vi "HFRR ADV v04 new software.vi"() -> ()   [LabVIEW 2025] (continued)
                  n3123 = local write "S 98"(w4157) -> ()
                }
                frame 97 {
                  n3124 = local write "S 99"(w4158) -> ()
                }
                frame 98 {
                  n3125 = local write "S 100"(w4159) -> ()
                }
                frame 99 {
                  n3126 = local write "S 101"(w4160) -> ()
                }
                frame 100 {
                  n3127 = local write "S 102"(w4161) -> ()
                }
                frame 101 {
                  n3128 = local write "S 103"(w4162) -> ()
                }
                frame 102 {
                  n3129 = local write "S 104"(w4163) -> ()
                }
                frame 103 {
                  n3130 = local write "S 105"(w4164) -> ()
                }
                frame 104 {
                  n3131 = local write "S 106"(w4165) -> ()
                }
                frame 105 {
                }
                frame 106 {
                  n3132 = property on="OK Button 17" class="Bool (strict)"("Boolean Text.Text"=w4166) -> ()  [unwired: 2 in, 2 out]
                }
                frame 107 {
                  n3133 = property on="OK Button 16" class="Bool (strict)"("Boolean Text.Text"=w4167) -> ()  [unwired: 2 in, 2 out]
                }
                frame 108 {
                  n3134 = property on="TITTLE" class="Str"("Caption.Text"=w4168) -> ()  [unwired: 2 in, 2 out]
                }
                frame 109 {
                  "String 30" <- w4169
                }
                frame 110 {
                  n3135 = property on="Test Date" class="Str"("Caption.Text"=w4170) -> ()  [unwired: 2 in, 2 out]
                  "String 31" <- w4170
                }
                frame 111 {
                  n3136 = property on="Sample ID" class="Str"("Caption.Text"=w4171) -> ()  [unwired: 2 in, 2 out]
                  "String 32" <- w4171
                }
                frame 112 {
                  n3137 = property on="Tested by" class="Str"("Caption.Text"=w4172) -> ()  [unwired: 2 in, 2 out]
                  "String 33" <- w4172
                }
                frame 113 {
                  n3138 = property on="System Configured Printers 2" class="Arr (strict)"("Caption.Text"=w4173) -> ()  [unwired: 2 in, 2 out]
                }
                frame 114 {
                  n3139 = property on="Selected Printer" class="Str"("Caption.Text"=w4174) -> ()  [unwired: 2 in, 2 out]
                }
                frame 115 {
                  n3140 = property on="Select Printer 3" class="DigNum (strict)"("Caption.Text"=w4175) -> ()  [unwired: 2 in, 2 out]
                }
                frame 116 {
                  n3141 = property on="Print" class="Bool (strict)"("Boolean Text.Text"=w4176) -> ()  [unwired: 2 in, 2 out]
                }
                frame 117 {
                  "String 41" <- w4177
                }
                frame 118 {
                  n3142 = property on="tested by" class="Str"("Caption.Text"=w4178) -> ()  [unwired: 2 in, 2 out]
                }
                frame 119 {
                }
                frame 120 {
                  n3143 = property on="Export" class="Bool (strict)"("Boolean Text.Text"=w4179) -> ()  [unwired: 2 in, 2 out]
                }
                frame 121 {
                  n3144 = property on="TEMP INTERCEPT:" class="DigNum (strict)"("Caption.Text"=w4180) -> ()  [unwired: 2 in, 2 out]
                }
                frame 122 {
                  n3145 = property on="AIR TEMP INTERCEPT:" class="DigNum (strict)"("Caption.Text"=w4181) -> ()  [unwired: 2 in, 2 out]
                }
                frame 123 {
                  n3146 = property on="Select File Type" class="Enum (strict)"("Caption.Text"=w4182) -> ()  [unwired: 2 in, 2 out]
                }
                frame 124 {
                  n3147 = property on="s.NO" class="Str"("Caption.Text"=w4183) -> ()  [unwired: 2 in, 2 out]
                  "String 45" <- w4183
                }
                frame 125 {
                  n3148 = property on="trip1 8" class="Bool (strict)"("Boolean Text.Text"=w4184) -> ()  [unwired: 2 in, 2 out]
                }
                frame 126, Default {
                }
              }
            }
          }
          frame #1 {
            w4192 = TRUE ("Visible")
            n3149 = local read "S 91"() -> (w4209:string)
            n3150 = local read "S 90"() -> (w4208:string)
            n3151 = local read "S 88"() -> (w4207:string)
            n3152 = property on="File Path" class="Path"("Caption.Text"=w4208) -> ()  [unwired: 2 in, 2 out]
            n3153 = property on="SrvM CP" class="Bool (strict)"("Boolean Text.Text"=w4207) -> ()  [unwired: 2 in, 2 out]
            n3154 = local read "S 71"() -> (w4202:string)
            n3155 = local read "S 86"() -> (w4204:string)
            n3156 = local read "S 85"() -> (w4205:string)
            n3157 = local read "S 87"() -> (w4203:string)
            n3158 = local read "S 84"() -> (w4206:string)
            n3159 = local read "S 103"() -> (w4191:string)
            n3160 = local read "S 104"() -> (w4190:string)
            n3161 = property on="ENTER THE NEW PASSWORD" class="Str"("Caption.Text"=w4203) -> ()  [unwired: 2 in, 2 out]
            n3162 = property on="Password" class="Str"("Caption.Text"=w4205) -> ()  [unwired: 2 in, 2 out]
            n3163 = property on="ENTER CURRENT PASSWORD" class="Str"("Caption.Text"=w4204) -> ()  [unwired: 2 in, 2 out]
            n3164 = property on="EDIT" class="Bool (strict)"("Boolean Text.Text"=w4202) -> ()  [unwired: 2 in, 2 out]
            n3165 = property on="SAVE" class="Bool (strict)"("Boolean Text.Text"=w4206) -> ()  [unwired: 2 in, 2 out]
            n3166 = Build Array(w4191, w4190) -> (w4189:string[])
            n3167 = property on="Heater Button" class="Bool (strict)"("Strings [4]"=w4189) -> ()  [unwired: 2 in, 2 out]
            n3168 = property on="CH-HUMIDITY WET" class="DigNum (strict)"("Caption.Size to Text?"=w4192) -> ()  [unwired: 2 in, 2 out]
            n3169 = property on="CH-HUMIDITY DRY" class="DigNum (strict)"("Caption.Size to Text?"=w4192) -> ()  [unwired: 2 in, 2 out]
            n3170 = property on="CH-POWER -" class="DigNum (strict)"("Caption.Size to Text?"=w4192) -> ()  [unwired: 2 in, 2 out]
            n3171 = property on="CH-HEATER" class="DigNum (strict)"("Caption.Size to Text?"=w4192) -> ()  [unwired: 2 in, 2 out]
            n3172 = property on="CH-POWER +" class="DigNum (strict)"("Caption.Size to Text?"=w4192) -> ()  [unwired: 2 in, 2 out]
            n3173 = local read "S 92"() -> (w4201:string)
            n3174 = local read "S 93"() -> (w4200:string)
            n3175 = local read "S 105"() -> (w4187:string)
            n3176 = local read "S 106"() -> (w4186:string)
            n3177 = Build Array(w4201, w4200) -> ()  [unwired: 1 out]
            n3178 = Build Array(w4187, w4186) -> (w4188:string[])
            n3179 = local read "S 95"() -> (w4198:string)
            n3180 = local read "S 94"() -> (w4199:string)
            n3181 = local read "bs"() -> (w4214:string)
            n3182 = local read "as"() -> (w4215:string)
            n3183 = property on="Humidity" class="Bool (strict)"("Strings [4]"=w4188) -> ()  [unwired: 2 in, 2 out]
            n3184 = Concatenate Strings(w4214, "\r", w4215) -> ()  [unwired: 1 out]
            n3185 = property on="STROKE GAIN :" class="DigNum (strict)"("Caption.Text"=w4198) -> ()  [unwired: 2 in, 2 out]
            n3186 = property on="DISPLACEMENT :" class="DigNum (strict)"("Caption.Text"=w4199) -> ()  [unwired: 2 in, 2 out]
            n3187 = property on="Rh After" class="DigNum (strict)"("Caption.Size to Text?"=TRUE ("Caption.Size to Text")) -> ()  [unwired: 2 in, 2 out]
            n3188 = local read "S 48"() -> (w4238:string)
            n3189 = local read "S 50"() -> (w4236:string)
            n3190 = local read "S 51"() -> (w4235:string)
            n3191 = local read "S 49"() -> (w4237:string)
            n3192 = local read "S 52"() -> (w4234:string)
            n3193 = local read "as"() -> (w4219:string)
            n3194 = local read "bs"() -> (w4220:string)
            n3195 = local read "S 56"() -> (w4233:string)
            n3196 = local read "S 57"() -> (w4232:string)
            n3197 = local read "S 58"() -> (w4231:string)
            n3198 = local read "S 59"() -> (w4230:string)
            n3199 = property on="OPEN" class="Bool (strict)"("Boolean Text.Text"=w4234) -> ()  [unwired: 2 in, 2 out]
            n3200 = property on="OPEN 1" class="Bool (strict)"("Boolean Text.Text"=w4238) -> ()  [unwired: 2 in, 2 out]
            n3201 = property on="OPEN 2" class="Bool (strict)"("Boolean Text.Text"=w4237) -> ()  [unwired: 2 in, 2 out]
            n3202 = property on="OPEN 3" class="Bool (strict)"("Boolean Text.Text"=w4236) -> ()  [unwired: 2 in, 2 out]
            n3203 = property on="OPEN 4" class="Bool (strict)"("Boolean Text.Text"=w4235) -> ()  [unwired: 2 in, 2 out]
            n3204 = Concatenate Strings(w4220, "\r", w4219) -> ()  [unwired: 1 out]
            n3205 = local read "S 102"() -> (w4193:string)
            n3206 = property on="КОФ1" class="DigNum (strict)"("Caption.Text"=w4233) -> ()  [unwired: 2 in, 2 out]
            n3207 = local read "S 98"() -> (w4197:string)
            n3208 = local read "S 99"() -> (w4196:string)
            n3209 = local read "S 100"() -> (w4195:string)
            n3210 = local read "S 101"() -> (w4194:string)
            n3211 = property on="КОФ2" class="DigNum (strict)"("Caption.Text"=w4232) -> ()  [unwired: 2 in, 2 out]
            n3212 = property on="КОФ3" class="DigNum (strict)"("Caption.Text"=w4231) -> ()  [unwired: 2 in, 2 out]
            n3213 = property on="КОФ4" class="DigNum (strict)"("Caption.Text"=w4230) -> ()  [unwired: 2 in, 2 out]
            n3214 = local read "bs"() -> (w4218:string)
            n3215 = local read "as"() -> (w4217:string)
            n3216 = property on="CH-POWER +" class="DigNum (strict)"("Caption.Text"=w4197) -> ()  [unwired: 2 in, 2 out]
            n3217 = property on="CH-POWER -" class="DigNum (strict)"("Caption.Text"=w4196) -> ()  [unwired: 2 in, 2 out]
            n3218 = property on="CH-HEATER" class="DigNum (strict)"("Caption.Text"=w4195) -> ()  [unwired: 2 in, 2 out]
            n3219 = property on="CH-HUMIDITY DRY" class="DigNum (strict)"("Caption.Text"=w4194) -> ()  [unwired: 2 in, 2 out]
            n3220 = property on="CH-HUMIDITY WET" class="DigNum (strict)"("Caption.Text"=w4193) -> ()  [unwired: 2 in, 2 out]
            n3221 = local read "S 60"() -> (w4229:string)
            n3222 = local read "S 54"() -> (w4239:string)
            n3223 = Concatenate Strings(w4218, "\r", w4217) -> ()  [unwired: 1 out]
            n3224 = Concatenate Strings(w4239, w4229) -> ()  [unwired: 1 out]
            n3225 = local read "S 77"() -> (→"String 43":string)
            n3226 = local read "S 76"() -> (w4212:string)
            n3227 = local read "S 78"() -> (w4211:string)
            n3228 = local read "S 71"() -> (w4223:string)
            n3229 = local read "S 66"() -> (w4228:string)
            n3230 = local read "S 67"() -> (w4227:string)
            n3231 = local read "S 68"() -> (w4226:string)
            n3232 = local read "S 69"() -> (w4225:string)
            n3233 = local read "S 70"() -> (w4224:string)
            n3234 = property on="AIR TEMP" class="DigNum (strict)"("Caption.Text"=w4211) -> ()  [unwired: 2 in, 2 out]
            n3235 = property on="Set Strk" class="DigNum (strict)"("Caption.Text"=w4212) -> ()  [unwired: 2 in, 2 out]
            n3236 = property on="FRIC. FORCE :" class="DigNum (strict)"("Caption.Text"=w4228) -> ()  [unwired: 2 in, 2 out]
            n3237 = property on="TEMPERATURE :" class="DigNum (strict)"("Caption.Text"=w4227) -> ()  [unwired: 2 in, 2 out]
            n3238 = property on="SPEED OUT:" class="DigNum (strict)"("Caption.Text"=w4226) -> ()  [unwired: 2 in, 2 out]
            n3239 = property on="AIR TEMPERATURE :" class="DigNum (strict)"("Caption.Text"=w4225) -> ()  [unwired: 2 in, 2 out]
            n3240 = property on="HUMIDITY:" class="DigNum (strict)"("Caption.Text"=w4224) -> ()  [unwired: 2 in, 2 out]
            n3241 = property on="EDIT" class="Bool (strict)"("Boolean Text.Text"=w4223) -> ()  [unwired: 2 in, 2 out]
            n3242 = local read "S 79"() -> (w4210:string)
          }
          frame #2 {
          }
        }
        n3243 = local write "Lan flag"(10.0 ("Lan flag")) -> ()
      }
      frame Enabled {
      }
    }
    n3244 = Wait (ms)(milliseconds to wait=u32 2000) -> ()  [unwired: 1 out]
    n3245 = local read "Quit"() -> (w4013:bool)
  }
  n3246 = disable-structure shown="Disabled" {
    frame Disabled {
      n3247 = while {
        tunnel: [w4241] -> _
        i -> [w4241]
        stop <- w4240 continue-if-true
        n3248 = Wait (ms)(milliseconds to wait=u32 50) -> ()  [unwired: 1 out]
        n3249 = stacked-sequence {
          frame #0 {
            # "Controls Text color"
            # "Controls BG color"
            n3250 = property on="FILE" class="Str"("Text.Text Colors:Text Color"="SC  Text") -> ()  [unwired: 2 in, 2 out]
            n3251 = property on="Fuel Discription :" class="Str"("Text.Text Colors:Text Color"="SC  Text") -> ()  [unwired: 2 in, 2 out]
            n3252 = property on="tested by" class="Str"("Text.Text Colors:Text Color"="SC  Text") -> ()  [unwired: 2 in, 2 out]
            n3253 = property on="Remarks :" class="Str"("Text.Text Colors:Text Color"="SC  Text") -> ()  [unwired: 2 in, 2 out]
            n3254 = property class="DigNum (strict)"("Numeric Text.Text Colors:BG Color"="NC BG") -> ()  [unwired: 2 in, 2 out]
            n3255 = property class="DigNum (strict)"("Numeric Text.Text Colors:BG Color"="NC BG") -> ()  [unwired: 2 in, 2 out]
            n3256 = property class="DigNum (strict)"("Numeric Text.Text Colors:BG Color"="NC BG") -> ()  [unwired: 2 in, 2 out]
            n3257 = property class="DigNum (strict)"("Numeric Text.Text Colors:BG Color"="NC BG") -> ()  [unwired: 2 in, 2 out]
            n3258 = property class="DigNum (strict)"("Numeric Text.Text Colors:BG Color"="NC BG") -> ()  [unwired: 2 in, 2 out]
            n3259 = property class="DigNum (strict)"("Numeric Text.Text Colors:BG Color"="NC BG") -> ()  [unwired: 2 in, 2 out]
            n3260 = property class="DigNum (strict)"("Numeric Text.Text Colors:BG Color"="NC BG") -> ()  [unwired: 2 in, 2 out]
            n3261 = property class="DigNum (strict)"("Numeric Text.Text Colors:BG Color"="NC BG") -> ()  [unwired: 2 in, 2 out]
            n3262 = property class="DigNum (strict)"("Numeric Text.Text Colors:BG Color"="NC BG") -> ()  [unwired: 2 in, 2 out]
            n3263 = property class="DigNum (strict)"("Numeric Text.Text Colors:BG Color"="NC BG") -> ()  [unwired: 2 in, 2 out]
            n3264 = property class="DigNum (strict)"("Numeric Text.Text Colors:BG Color"="NC BG") -> ()  [unwired: 2 in, 2 out]
            n3265 = property class="DigNum (strict)"("Numeric Text.Text Colors:BG Color"="NC BG") -> ()  [unwired: 2 in, 2 out]
            n3266 = property on="FILE" class="Str"("Text.Text Colors:BG Color"="SC BG 3") -> ()  [unwired: 2 in, 2 out]
            n3267 = property on="Fuel Discription :" class="Str"("Text.Text Colors:BG Color"="SC BG 3") -> ()  [unwired: 2 in, 2 out]
            n3268 = property on="tested by" class="Str"("Text.Text Colors:BG Color"="SC BG 3") -> ()  [unwired: 2 in, 2 out]
            n3269 = property on="Remarks :" class="Str"("Text.Text Colors:BG Color"="SC BG 3") -> ()  [unwired: 2 in, 2 out]
            n3270 = property class="DigNum (strict)"("Numeric Text.Text Colors:Text Color"="NC Text") -> ()  [unwired: 2 in, 2 out]
            n3271 = property class="DigNum (strict)"("Numeric Text.Text Colors:Text Color"="NC Text") -> ()  [unwired: 2 in, 2 out]
            n3272 = property class="DigNum (strict)"("Numeric Text.Text Colors:Text Color"="NC Text") -> ()  [unwired: 2 in, 2 out]
            n3273 = property class="DigNum (strict)"("Numeric Text.Text Colors:Text Color"="NC Text") -> ()  [unwired: 2 in, 2 out]
            n3274 = property class="DigNum (strict)"("Numeric Text.Text Colors:Text Color"="NC Text") -> ()  [unwired: 2 in, 2 out]
            n3275 = property class="DigNum (strict)"("Numeric Text.Text Colors:Text Color"="NC Text") -> ()  [unwired: 2 in, 2 out]
            n3276 = property class="DigNum (strict)"("Numeric Text.Text Colors:Text Color"="NC Text") -> ()  [unwired: 2 in, 2 out]
            n3277 = property class="DigNum (strict)"("Numeric Text.Text Colors:Text Color"="NC Text") -> ()  [unwired: 2 in, 2 out]
            n3278 = property class="DigNum (strict)"("Numeric Text.Text Colors:Text Color"="NC Text") -> ()  [unwired: 2 in, 2 out]
            n3279 = property class="DigNum (strict)"("Numeric Text.Text Colors:Text Color"="NC Text") -> ()  [unwired: 2 in, 2 out]
            n3280 = property class="DigNum (strict)"("Numeric Text.Text Colors:Text Color"="NC Text") -> ()  [unwired: 2 in, 2 out]
            n3281 = property class="DigNum (strict)"("Numeric Text.Text Colors:Text Color"="NC Text") -> ()  [unwired: 2 in, 2 out]
            n3282 = property class="DigNum (strict)"("Numeric Text.Text Colors:Text Color"="NI Text  2") -> ()  [unwired: 2 in, 2 out]
            n3283 = property class="DigNum (strict)"("Numeric Text.Text Colors:Text Color"="NI Text  2") -> ()  [unwired: 2 in, 2 out]
            n3284 = property class="DigNum (strict)"("Numeric Text.Text Colors:Text Color"="NI Text  2") -> ()  [unwired: 2 in, 2 out]
            n3285 = property class="DigNum (strict)"("Numeric Text.Text Colors:Text Color"="NI Text  2") -> ()  [unwired: 2 in, 2 out]
            n3286 = property class="DigNum (strict)"("Numeric Text.Text Colors:Text Color"="NI Text  2") -> ()  [unwired: 2 in, 2 out]
            n3287 = property class="DigNum (strict)"("Numeric Text.Text Colors:Text Color"="NI Text  2") -> ()  [unwired: 2 in, 2 out]
            n3288 = property class="DigNum (strict)"("Numeric Text.Text Colors:Text Color"="NI Text  2") -> ()  [unwired: 2 in, 2 out]
            n3289 = property class="DigNum (strict)"("Numeric Text.Text Colors:Text Color"="NI Text  2") -> ()  [unwired: 2 in, 2 out]
            n3290 = property class="DigNum (strict)"("Numeric Text.Text Colors:Text Color"="NI Text  2") -> ()  [unwired: 2 in, 2 out]
            n3291 = property class="DigNum (strict)"("Numeric Text.Text Colors:Text Color"="NI Text  2") -> ()  [unwired: 2 in, 2 out]
            n3292 = property class="DigNum (strict)"("Numeric Text.Text Colors:Text Color"="NI Text  2") -> ()  [unwired: 2 in, 2 out]
            n3293 = property class="DigNum (strict)"("Numeric Text.Text Colors:Text Color"="NI Text  2") -> ()  [unwired: 2 in, 2 out]
            n3294 = property class="DigNum (strict)"("Numeric Text.Text Colors:Text Color"="NI Text  2") -> ()  [unwired: 2 in, 2 out]
            n3295 = property class="DigNum (strict)"("Numeric Text.Text Colors:Text Color"="NI Text  2") -> ()  [unwired: 2 in, 2 out]
            n3296 = property class="DigNum (strict)"("Numeric Text.Text Colors:Text Color"="NI Text  2") -> ()  [unwired: 2 in, 2 out]
            n3297 = property on="Coefficient Of Friction" class="XYGraph (strict)"("Plot Area:Colors:FG Color"="GFG  2", "Plot Area:Colors:BG Color"="GBG   2") -> ()  [unwired: 2 in, 2 out]
            n3298 = property on="Humidity ( %RH )" class="XYGraph (strict)"("Plot Area:Colors:FG Color"="GFG  2", "Plot Area:Colors:BG Color"="GBG   2") -> ()  [unwired: 2 in, 2 out]
            n3299 = property on="Air Temperature  ( °C )" class="XYGraph (strict)"("Plot Area:Colors:FG Color"="GFG  2", "Plot Area:Colors:BG Color"="GBG   2") -> ()  [unwired: 2 in, 2 out]
            n3300 = property on="Sample Temperature ( °C )" class="XYGraph (strict)"("Plot Area:Colors:FG Color"="GFG  2", "Plot Area:Colors:BG Color"="GBG   2") -> ()  [unwired: 2 in, 2 out]
            n3301 = property class="DigNum (strict)"("Numeric Text.Text Colors:BG Color"="NI BG 2") -> ()  [unwired: 2 in, 2 out]
            n3302 = property class="DigNum (strict)"("Numeric Text.Text Colors:BG Color"="NI BG 2") -> ()  [unwired: 2 in, 2 out]
            n3303 = property class="DigNum (strict)"("Numeric Text.Text Colors:BG Color"="NI BG 2") -> ()  [unwired: 2 in, 2 out]
            n3304 = property class="DigNum (strict)"("Numeric Text.Text Colors:BG Color"="NI BG 2") -> ()  [unwired: 2 in, 2 out]
            n3305 = property class="DigNum (strict)"("Numeric Text.Text Colors:BG Color"="NI BG 2") -> ()  [unwired: 2 in, 2 out]
            n3306 = property class="DigNum (strict)"("Numeric Text.Text Colors:BG Color"="NI BG 2") -> ()  [unwired: 2 in, 2 out]
            n3307 = property class="DigNum (strict)"("Numeric Text.Text Colors:BG Color"="NI BG 2") -> ()  [unwired: 2 in, 2 out]
            n3308 = property class="DigNum (strict)"("Numeric Text.Text Colors:BG Color"="NI BG 2") -> ()  [unwired: 2 in, 2 out]
            n3309 = property class="DigNum (strict)"("Numeric Text.Text Colors:BG Color"="NI BG 2") -> ()  [unwired: 2 in, 2 out]
            n3310 = property class="DigNum (strict)"("Numeric Text.Text Colors:BG Color"="NI BG 2") -> ()  [unwired: 2 in, 2 out]
            n3311 = property class="DigNum (strict)"("Numeric Text.Text Colors:BG Color"="NI BG 2") -> ()  [unwired: 2 in, 2 out]
            n3312 = property class="DigNum (strict)"("Numeric Text.Text Colors:BG Color"="NI BG 2") -> ()  [unwired: 2 in, 2 out]
            n3313 = property class="DigNum (strict)"("Numeric Text.Text Colors:BG Color"="NI BG 2") -> ()  [unwired: 2 in, 2 out]
            n3314 = property class="DigNum (strict)"("Numeric Text.Text Colors:BG Color"="NI BG 2") -> ()  [unwired: 2 in, 2 out]
            n3315 = property class="DigNum (strict)"("Numeric Text.Text Colors:BG Color"="NI BG 2") -> ()  [unwired: 2 in, 2 out]
            n3316 = property class="Bool"("Colors [4]"="Boolean BC T & BG") -> ()  [unwired: 2 in, 2 out]
            n3317 = property on="Save & Continue" class="Bool (strict)"("Colors [4]"="Boolean BC T & BG") -> ()  [unwired: 2 in, 2 out]
            n3318 = property on="Heater Button" class="Bool (strict)"("Colors [4]"="Boolean BC T & BG") -> ()  [unwired: 2 in, 2 out]
            n3319 = property class="Bool"("Colors [4]"="Boolean BC T & BG") -> ()  [unwired: 2 in, 2 out]
            n3320 = property on="Humidity" class="Bool (strict)"("Colors [4]"="Boolean BC T & BG") -> ()  [unwired: 2 in, 2 out]
            n3321 = property class="Bool (strict)"("Colors [4]"="Boolean BC T & BG") -> ()  [unwired: 2 in, 2 out]
            n3322 = property on="RUN" class="Bool (strict)"("Colors [4]"="Boolean BC T & BG") -> ()  [unwired: 2 in, 2 out]
            n3323 = property on="trip1 8" class="Bool (strict)"("Colors [4]"="Boolean BC T & BG") -> ()  [unwired: 2 in, 2 out]
            n3324 = property class="Bool"("Colors [4]"="Boolean BC T & BG") -> ()  [unwired: 2 in, 2 out]
            n3325 = property class="Bool (strict)"("Colors [4]"="Boolean BC T & BG") -> ()  [unwired: 2 in, 2 out]
            n3326 = property on="OPEN 1" class="Bool (strict)"("Colors [4]"="Boolean BC T & BG 2") -> ()  [unwired: 2 in, 2 out]
            n3327 = property on="OPEN 2" class="Bool (strict)"("Colors [4]"="Boolean BC T & BG 2") -> ()  [unwired: 2 in, 2 out]
            n3328 = property on="OPEN 3" class="Bool (strict)"("Colors [4]"="Boolean BC T & BG 2") -> ()  [unwired: 2 in, 2 out]
            n3329 = property on="OPEN 4" class="Bool (strict)"("Colors [4]"="Boolean BC T & BG 2") -> ()  [unwired: 2 in, 2 out]
            n3330 = property on="OPEN" class="Bool (strict)"("Colors [4]"="Boolean BC T & BG 2") -> ()  [unwired: 2 in, 2 out]
            n3331 = property on="rstv2" class="Bool"("Colors [4]"="Boolean BC T & BG 2") -> ()  [unwired: 2 in, 2 out]
            n3332 = property on="RST CP" class="Bool"("Colors [4]"="Boolean BC T & BG 2") -> ()  [unwired: 2 in, 2 out]
            n3333 = property on="RSTV1 3" class="Bool"("Colors [4]"="Boolean BC T & BG 2") -> ()  [unwired: 2 in, 2 out]
            n3334 = property on="RSTV1 2" class="Bool"("Colors [4]"="Boolean BC T & BG 2") -> ()  [unwired: 2 in, 2 out]
          }
          frame #1 {
          }
        }
        n3335 = local read "Quit"() -> (w4240:bool)
      }
    }
    frame Enabled {
    }
  }
  n3336 = while {
    shift-right: [w4258] -> _
    shift-left: _ -> [w4259]
    shift-right: [w4256] -> _
    shift-left: T14 {"Read Heave and Surge"="", "Bytes at Heave Port"=0.0, "Heave and Surge COM Port:"="COM9", "Com Port 2"="COM7", "Residual Due"="", "Heave COM Status 2"=TRUE, "Heave COM Status"=TRUE, "Port 2"=TRUE, "Sway PPR"=6400.0, "Surge PPR"=6400.0, "Heave PPR"=6400.0, "Sway Pitch"=2.0, "Surge Pitch"=3.0, "Heave Pitch"=4.0, "Sway Pulses/mm"=320.0, "Surge Pulses/mm"=1600.0, "Heave Pulses/mm"=1600.0, "inner loop"=0.0, "Read Heave and Surge 2"="", "String 36"="", "Write S"=FALSE, "WriteCC1"=[""], "Heave COM Loop"=0, "LastCom"="", "EXIT"=FALSE, "Error Heave"={"status"=TRUE, "code"=-1073807343, "source"=""}} -> [w4255]
    shift-right: [w4253] -> _
    shift-left: enum16{"init", "MAIN", "Panel Close"}."init" -> [w4254]
    stop <- w4257 stop-if-true
    n3337 = case shown="\"init\"" w4254 {
      tunnel: w4259 -> [w4273 w4288 w4358 w4360]
      tunnel: [w4267 w4306 w4358 w4360] -> w4258
      tunnel: [_ _ TRUE _] -> w4257
      tunnel: [w4263 w4303 w4356 w4359] -> w4256
      tunnel: w4255 -> [w4270 w4287 w4356 w4359]
      tunnel: [enum16{"init", "MAIN", "Panel Close"}."MAIN" w4281 _ _] -> w4253
      frame "init" {
        n3338 = Bundle By Name(cluster=w4270, "Heave and Surge COM Port:"="C3 :") -> (w4269:T14)
        n3339 = call "Instrument fgv.vi"("Enum"=T24."INIT", "error in (no error) 2"=w4273, "INPUT"=w4269) -> ("error"=w4271:errorcluster, "output"=w4266:T14)  [unwired: 6 in, 1 out]
        n3340 = case shown="No Error" w4271 {
          selector: w4271 -> [w4275 _]
          tunnel: [w4275 w4279] -> w4267
          tunnel: w4266 -> [w4274 w4277]
          tunnel: [w4274 w4276] -> w4264
          frame No Error {
          }
          frame Error {
            n3341 = call "Instrument fgv.vi"("Enum"=T24."ERROR INIT", "INPUT"=w4277) -> ("error"=w4280:errorcluster, "output"=w4276:T14)  [unwired: 7 in, 1 out]
            n3342 = call <vilib>:"Clear Errors.vi"("error in (no error)"=w4280) -> ("error out"=w4279:errorcluster)  [unwired: 5 in, 1 out]
          }
        }
        n3343 = local read "LastCom"() -> (w4262:string)
        n3344 = Unbundle By Name(w4264) -> ("Heave COM Status 2"=→"COM Status" →"Instrument Status":bool, "Error Heave"=→"Error":errorcluster)  [unwired: 1 out]
        n3345 = Bundle By Name(cluster=w4264, "LastCom"=w4262) -> (w4263:T14)
      }
      frame "MAIN" {
        n3346 = Unbundle By Name(w4287) -> ("Com Port 2"=w4308:refnum<visa-resource-name>)
        n3347 = local write "Com Port 4"(w4308) -> ()
        n3348 = local read "C3 :"() -> (w4285:refnum<visa-resource-name>)
        n3349 = Divide(x="Heave PPR", y="Heave Pitch") -> (x/y=→"Heave Pulses/mm":dbl)
        n3350 = Bundle By Name(cluster=w4287, "Heave and Surge COM Port:"=w4285) -> (w4286:T14)
        n3351 = Equal?(x=w4308, y=w4285) -> (x = y?=w4307:bool)
        n3352 = Divide(x="Sway PPR", y="Sway Pitch") -> (x/y=→"Sway Pulses/mm":dbl)
        n3353 = case shown="False" w4307 {
          tunnel: [w4312 w4329] -> w4306
          tunnel: w4288 -> [w4313 w4335]
          tunnel: w4286 -> [w4311 w4333]
          tunnel: [w4310 w4328] -> w4303
          frame False {
            n3354 = call <vilib>:"Clear Errors.vi"("error in (no error)"=w4313) -> ("error out"=w4309:errorcluster)  [unwired: 5 in, 1 out]
            n3355 = call "Instrument fgv.vi"("Enum"=T24."ERROR INIT", "error in (no error) 2"=w4309, "INPUT"=w4311) -> ("error"=w4315:errorcluster, "output"=w4310:T14)  [unwired: 6 in, 1 out]
            n3356 = call <vilib>:"Clear Errors.vi"("error in (no error)"=w4315) -> ("error out"=w4312:errorcluster)  [unwired: 5 in, 1 out]
          }
          frame True {
            n3357 = call "Instrument fgv.vi"("Enum"=T24."READ", "error in (no error) 2"=w4335, "INPUT"=w4333) -> ("error"=w4334:errorcluster, "output"=w4325:T14)  [unwired: 6 in, 1 out]
            n3358 = Bundle By Name(cluster=w4325, "String 36"="String 11") -> (w4324:T14)
            n3359 = case shown="True" "Write S" {
              selector: "Write S" -> [_ w4355]
              tunnel: w4334 -> [w4348 w4354]
              tunnel: [w4348 w4353] -> w4321
              tunnel: w4324 -> [w4347 w4350]
              tunnel: [w4347 w4349] -> w4320
              frame False {
              }
              frame True {
                n3360 = Not(x=w4355) -> (.not. x?=w4351:bool)
                n3361 = local write "Write S"(w4351) -> ()
                n3362 = call "Instrument fgv.vi"("Enum"=T24."MANUAL WRITE", "error in (no error) 2"=w4354, "INPUT"=w4350) -> ("error"=w4353:errorcluster, "output"=w4349:T14)  [unwired: 6 in, 1 out]
              }
            }
            n3363 = Array Size(array="WriteHumidity") -> (size(s)=w4318:i32)
            n3364 = Greater Than 0?(x=w4318) -> (x > 0?=w4316:bool)
            n3365 = call "Instrument fgv.vi"("Enum"=T24."WRITE", "error in (no error) 2"=w4321, "WriteCC1"="WriteHumidity", "INPUT"=w4320) -> ("error"=w4331:errorcluster, "WriteCC1 2"=w4319:string[], "output"=w4330:T14)  [unwired: 5 in]
            n3366 = case shown="True" w4316 {
              tunnel: w4319 -> [_ w4337]
              frame False {
              }
              frame True {
                n3367 = local write "WriteHumidity"(w4337) -> ()
              }
            }
            n3368 = case shown="Error" w4331 {
              selector: w4331 -> [w4338 w4341]
              tunnel: w4330 -> [w4339 w4346]
              tunnel: [w4339 w4345] -> w4328
              tunnel: [w4338 w4343] -> w4329
              frame No Error {
              }
              frame Error {
                n3369 = call <vilib>:"Clear Errors.vi"("error in (no error)"=w4341) -> ("error out"=w4340:errorcluster)  [unwired: 5 in, 1 out]
                n3370 = call "Instrument fgv.vi"("Enum"=T24."ERROR INIT", "error in (no error) 2"=w4340, "INPUT"=w4346) -> ("error"=w4344:errorcluster, "output"=w4345:T14)  [unwired: 6 in, 1 out]
                n3371 = call <vilib>:"Clear Errors.vi"("error in (no error)"=w4344) -> ("error out"=w4343:errorcluster)  [unwired: 5 in, 1 out]
              }
            }
            n3372 = Unbundle By Name(w4328) -> ("LastCom"=→"LastCom":string, "Read Heave and Surge"=→"Read Humidity":string)
          }
        }
        n3373 = Divide(x="Surge PPR", y="Surge Pitch") -> (x/y=→"Surge Pulses/mm":dbl)
        n3374 = Unbundle By Name(w4303) -> ("Heave COM Status 2"=w4305:bool, "Heave COM Status"=w4304:bool, "Error Heave"=w4301:errorcluster, "Bytes at Heave Port"=→"Bytes at Humidity Port":dbl)
        n3375 = Unbundle By Name(w4301) -> ("status"=→"Humidity Port":bool)
        n3376 = Not(x=w4304) -> (.not. x?=w4289:bool)
        n3377 = local write "Error"(w4301) -> ()
        n3378 = Not(x=w4305) -> (.not. x?=w4290:bool)
        n3379 = local write "Instrument Status"(w4289) -> ()
        n3380 = local write "COM Status"(w4290) -> ()
        n3381 = local read "Quit"() -> (w4282:bool)
        n3382 = Select(t=enum16{"init", "MAIN", "Panel Close"}."Panel Close", s=w4282, f=enum16{"init", "MAIN", "Panel Close"}."MAIN") -> (s? t:f=w4281:enum16{"init", "MAIN", "Panel Close"})
      }
      frame "Panel Close" {
      }
      frame Default {
      }
    }
  }
  n3383 = while {
    stop <- w4386 stop-if-true
    n3384 = local read "Read Humidity"() -> (w4367:string)
    n3385 = call <vilib>:"High Resolution Polling Wait.vi"("seconds to wait"=0.1) -> ()  [unwired: 10 in, 1 out]
    n3386 = Spreadsheet String To Array(delimiter (Tab)=",", format string="", spreadsheet string=w4367, array type (2D Dbl)=string[] []) -> (array=w4381:string[])
    n3387 = for {
      tunnel: w4381 -> [w4391] mode=indexing
      tunnel: string[] ["STATE;", "SET;", "RH;", "T;", "AMB_RH;", "AMB_T;", "PUMP;", "FAN_IN;", "FAN_OUT;", "DEHUM;", "CURRENT;", "STALL;"] -> [w4390] mode=indexing
      tunnel: [w4389] -> w4380 mode=indexing
      n3388 = Match Pattern(string=w4391, regular expression=w4390) -> (after substring=w4389:string)  [unwired: 1 in, 3 out]
    }
    n3389 = Index Array(array=w4380) -> (element #1=→"STATE :":string, element #2=→"SET :":string, element #3=w4369:string, element #4=→"T :":string, element #5=w4366:string, element #6=→"AMB_T :":string, element #7=→"PUMP :":string, element #8=→"FAN_IN :":string, element #9=→"FAN_OUT :":string, element #10=→"DEHUM :":string, element #11=→"CURRENT :":string, element #12=→"STALL :":string)  [unwired: 12 in]
    "RH :" <- w4369
    "AMB_RH :" <- w4366
    n3390 = Fract/Exp String To Number(string=w4369) -> (number=w4361:dbl)  [unwired: 3 in, 1 out]
    n3391 = Fract/Exp String To Number(string=w4366) -> (number=w4365:dbl)  [unwired: 3 in, 1 out]
    n3392 = local write "Ambient Humidity :"(w4365) -> ()
    n3393 = Equal?(x=w4361, y=0.0) -> (x = y?=w4363:bool)
    n3394 = case shown="True" w4363 {
      tunnel: [w4387 w4388] -> w4362
      tunnel: w4361 -> [w4387 _]
      frame False {
        (unwired) 0.0
        "Humidity temp" <- w4387
      }
      frame True {
        n3395 = local read "Humidity temp"() -> (w4388:dbl)
      }
    }
    "RH Numeric:" <- w4362
    n3396 = local read "Quit"() -> (w4386:bool)
  }
  n3397 = disable-structure shown="Disabled" {
    frame Disabled {
      n3398 = while {
        tunnel: [w4625] -> _
        i -> [w4625]
        stop <- w4622 stop-if-true
        n3399 = local read "powstat"() -> (w4623:bool)
        n3400 = case shown="True" w4623 {
          frame False {
          }
          frame True {
            n3401 = local read "RUN"() -> (w4626:bool)
            n3402 = case shown="True" w4626 {
              frame False {
                w4656 = 65.0 ("y")
                n3403 = local read "Set Hz"() -> (w4684:dbl)
                n3404 = local read "NORMAL LOAD"() -> (w4685:dbl)
                n3405 = Multiply(x=w4684, y=60.0) -> (x*y=w4691:dbl)
                n3406 = Multiply(x=1.2 ("y"), y=0.949) -> (x*y=w4660:dbl)
                n3407 = Multiply(x=1.2 ("y"), y=0.8166) -> (x*y=w4664:dbl)
                n3408 = Multiply(x=1.2 ("y"), y=0.851) -> (x*y=w4659:dbl)
                n3409 = local read "FF 2"() -> (w4683:dbl)
                n3410 = Absolute Value(x=w4691) -> (abs(x)=w4689:dbl)
                n3411 = case shown="13.." w4683 {
                  tunnel: [1 2 3] -> w4681
                  frame 0..10, Default {
                    # "Normal"
                  }
                  frame 11, 12 {
                  }
                  frame 13.. {
                  }
                }
                "FF STATE" <- w4681
                n3412 = local read "TEMP"() -> (w4644:dbl)
                n3413 = local read item#-1() -> (w4658)
                n3414 = Less?(x=w4658, y=w4664) -> (x < y?=w4661:bool)
                n3415 = In Range and Coerce(upper limit=w4660, x=w4658, lower limit=w4659) -> (In Range?=w4662:bool)  [unwired: 1 out]
                n3416 = case shown="3601.." w4689 {
                  tunnel: [1 2 3] -> w4687
                  frame 0..3000, Default {
                    # "Normal"
                  }
                  frame 3001..3600 {
                  }
                  frame 3601.. {
                  }
                }
                n3417 = case shown="11.." w4685 {
                  tunnel: [1 3] -> w4686
                  frame 1..10, Default {
                  }
                  frame 11.. {
                  }
                }
                "NL STATE" <- w4686
                n3418 = Multiply(x=1.2 ("y"), y=0.95) -> (x*y=w4674:dbl)
                n3419 = Multiply(x=w4656, y=0.954) -> (x*y=w4648:dbl)
                n3420 = Or(x=w4661, y=w4662) -> (x .or. y?=w4663:bool)
                n3421 = Greater Or Equal?(x=w4658, y=w4674) -> (x >= y?=w4671:bool)
                n3422 = Multiply(x=w4656, y=0.99) -> (x*y=w4645:dbl)
                n3423 = Greater Or Equal?(x=w4644, y=w4645) -> (x >= y?=w4650:bool)
                n3424 = Greater Or Equal?(x=w4644, y=w4648) -> (x >= y?=w4647:bool)
                n3425 = case shown="0, 1, Default" w4658 {
                  tunnel: [1 3] -> w4675
                  frame 0, 1, Default {
                  }
                  frame 2.. {
                  }
                }
                n3426 = case shown="True" w4671 {
                  tunnel: [1 3] -> w4676
                  frame False {
                  }
                  frame True {
                  }
                }
                n3427 = case shown="True" w4663 {
                  tunnel: [1 2] -> w4677
                  frame False {
                  }
                  frame True {
                  }
                }
                n3428 = case shown="..0" w4644 {
                  tunnel: [2 3 3 1] -> w4651
                  frame 61, 62 {
                  }
                  frame 63.. {
                  }
                  frame ..0 {
                  }
                  frame 10..60, Default {
                  }
                }
                n3429 = case shown="True" w4650 {
                  tunnel: [1 3] -> w4652
                  frame False {
                  }
                  frame True {
                  }
                }
                n3430 = Number To Decimal String(number=w4687) -> (decimal integer string=w4688:string)  [unwired: 1 in]
                n3431 = case shown="True" w4647 {
                  tunnel: [1 2] -> w4653
                  frame False {
                  }
                  frame True {
                  }
                }
                n3432 = Number To Decimal String(number=1) -> (decimal integer string=→"Air temp":string)  [unwired: 1 in]
                n3433 = Number To Decimal String(number=w4681) -> (decimal integer string=→"ff_st":string)  [unwired: 1 in]
                n3434 = local write "sp_st"(w4688) -> ()
                n3435 = Number To Decimal String(number=w4686) -> (decimal integer string=→"nl_st":string)  [unwired: 1 in]
                n3436 = Build Array(w4651, w4652, w4653) -> (w4654:i32[])
                n3437 = Build Array(w4675, w4676, w4677) -> (w4678:i32[])
                n3438 = Array Max & Min(array=w4654) -> (max value=w4655:i32)  [unwired: 3 out]
                n3439 = Array Max & Min(array=w4678) -> (max value=w4679:i32)  [unwired: 3 out]
                n3440 = Number To Decimal String(number=w4655) -> (decimal integer string=w4643:string)  [unwired: 1 in]
                n3441 = Number To Decimal String(number=w4679) -> (decimal integer string=→"Stroke Ln 2":string)  [unwired: 1 in]
                n3442 = local write "temp_st"(w4643) -> ()
              }
              frame True {
                w4741 = 65.0 ("y")
                # "Healthy -1\nWarning -2\nError -3"
                n3443 = local read "TEMP"() -> (w4752:dbl)
                n3444 = local read "NORMAL LOAD"() -> (w4756:dbl)
                n3445 = local read "Set Hz"() -> (w4754:dbl)
                n3446 = Multiply(x=1.2 ("y"), y=0.949) -> (x*y=w4736:dbl)
                n3447 = Multiply(x=1.2 ("y"), y=0.8166) -> (x*y=w4732:dbl)
                n3448 = Multiply(x=1.2 ("y"), y=0.851) -> (x*y=w4737:dbl)
                n3449 = Multiply(x=w4741, y=0.954) -> (x*y=w4748:dbl)
                n3450 = Multiply(x=w4741, y=0.99) -> (x*y=w4751:dbl)
                n3451 = Greater Or Equal?(x=w4752, y=w4751) -> (x >= y?=w4746:bool)
                n3452 = Multiply(x=w4754, y=60.0) -> (x*y=w4760:dbl)
                n3453 = Greater Or Equal?(x=w4752, y=w4748) -> (x >= y?=w4749:bool)
                n3454 = local read "FF 2"() -> (w4755:dbl)
                n3455 = local read item#-1() -> (w4738)
                n3456 = Less?(x=w4738, y=w4732) -> (x < y?=w4735:bool)
                n3457 = In Range and Coerce(upper limit=w4736, x=w4738, lower limit=w4737) -> (In Range?=w4734:bool)  [unwired: 1 out]
                n3458 = Absolute Value(x=w4760) -> (abs(x)=w4758:dbl)
                n3459 = case shown="63.." w4752 {
                  tunnel: [2 3 3 1] -> w4745
                  frame 61, 62 {
                  }
                  frame 63.. {
                  }
                  frame ..0 {
                  }
                  frame 10..60, Default {
                  }
                }
                n3460 = case shown="True" w4746 {
                  tunnel: [1 3] -> w4744
                  frame False {
                  }
                  frame True {
                  }
                }
                n3461 = case shown="True" w4749 {
                  tunnel: [1 2] -> w4743
                  frame False {
                  }
                  frame True {
                  }
                }
                n3462 = Multiply(x=1.2 ("y"), y=0.95) -> (x*y=w4722:dbl)
                n3463 = case shown="1..10, Default" w4756 {
                  tunnel: [1 3] -> w4763
                  frame 1..10, Default {
                  }
                  frame 11.. {
                  }
                }
                n3464 = case shown="0..10, Default" w4755 {
                  tunnel: [1 2 3] -> w4762
                  frame 0..10, Default {
                  }
                  frame 11, 12 {
                  }
                  frame 13.. {
                  }
                }
                n3465 = case shown="3601.." w4758 {
                  tunnel: [1 2 3] -> w4757
                  frame 0..3000, Default {
                    # "Normal"
                  }
                  frame 3001..3600 {
                  }
                  frame 3601.. {
                  }
                }
                n3466 = Or(x=w4735, y=w4734) -> (x .or. y?=w4733:bool)
                n3467 = Greater Or Equal?(x=w4738, y=w4722) -> (x >= y?=w4725:bool)
                n3468 = case shown="0, 1, Default" w4738 {
                  tunnel: [1 3] -> w4721
                  frame 0, 1, Default {
                  }
                  frame 2.. {
                  }
                }
                n3469 = case shown="True" w4725 {
                  tunnel: [1 3] -> w4720
                  frame False {
                  }
                  frame True {
                  }
                }
                n3470 = case shown="True" w4733 {
                  tunnel: [1 2] -> w4719
                  frame False {
                  }
                  frame True {
                  }
                }
                n3471 = Build Array(w4745, w4744, w4743) -> (w4742:i32[])
                n3472 = Number To Decimal String(number=w4757) -> (decimal integer string=→"sp_st":string)  [unwired: 1 in]
                n3473 = Array Max & Min(array=w4742) -> (max value=w4739:i32)  [unwired: 3 out]
                "TEMP STATE" <- w4739
                n3474 = Number To Decimal String(number=w4763) -> (decimal integer string=w4766:string)  [unwired: 1 in]
                n3475 = Number To Decimal String(number=w4762) -> (decimal integer string=w4764:string)  [unwired: 1 in]
                n3476 = Number To Decimal String(number=w4739) -> (decimal integer string=→"temp_st":string)  [unwired: 1 in]
                n3477 = Build Array(w4721, w4720, w4719) -> (w4718:i32[])
                n3478 = local write "nl_st"(w4766) -> ()
                n3479 = local write "ff_st"(w4764) -> ()
                n3480 = Number To Decimal String(number=1) -> (decimal integer string=w4761:string)  [unwired: 1 in]
                n3481 = Array Max & Min(array=w4718) -> (max value=w4717:i32)  [unwired: 3 out]
                n3482 = local write "Air temp"(w4761) -> ()
                n3483 = Number To Decimal String(number=w4717) -> (decimal integer string=w4716:string)  [unwired: 1 in]
                n3484 = local write "Stroke Ln 2"(w4716) -> ()
              }
            }
            n3485 = local read "Stroke Ln 2"() -> (w4628:string)
            n3486 = local read "nl_st"() -> (w4634:string)
            n3487 = local read "ff_st"() -> (w4631:string)
            n3488 = local read "sp_st"() -> (w4632:string)
            n3489 = local read "temp_st"() -> (w4633:string)
            n3490 = local read "Air temp"() -> (w4627:string)
            n3491 = Replace Array Subset(array="in", new element #1=w4634, index #1=1 ("index"), new element #2=w4631, index #2=2 ("index"), new element #3=w4633, index #3=3 ("index"), new element #4=w4632, index #4=4 ("index"), new element #5=w4628, index #5=5 ("index"), new element #6=w4627, index #6=6 ("index"), new element #7="Sensor State" ("new element/subarray"), index #7=0 ("index")) -> (→"out":string[])
          }
        }
        n3492 = Wait (ms)(milliseconds to wait=u32 10) -> ()  [unwired: 1 out]
        n3493 = local read "Quit"() -> (w4622:bool)
      }
      n3494 = while {
        stop <- w4597 stop-if-true
        n3495 = local read "run replace"() -> (w4599:bool)
        n3496 = Wait (ms)(milliseconds to wait=u32 100) -> ()  [unwired: 1 out]
        n3497 = Equal?(x="FLAG 2", y=0.0) -> (x = y?=w4600:bool)
        n3498 = case shown="True" w4600 {
          frame False {
          }
          frame True {
            n3499 = local write "FLAG 2"(100.0 ("FLAG 2")) -> ()
            n3500 = call <vilib>:"Read Characters From File.vi"("file path (dialog if empty)"=path "C:/LAB-IQ-NXT/WO 2449 TT.sig", "convert eol? (no:F)"=FALSE ("append to file? (new file:F)")) -> ("character string"=w4603:string)  [unwired: 4 in, 3 out]
            n3501 = call <vilib>:"Read Characters From File.vi"("file path (dialog if empty)"=path "C:/LAB-IQ-NXT/WO 2449 TRH.sig", "convert eol? (no:F)"=FALSE ("append to file? (new file:F)")) -> ("character string"=w4604:string)  [unwired: 4 in, 3 out]
            n3502 = Decimal String To Number(string=w4603) -> (number=w4605:i32)  [unwired: 2 in, 1 out]
            n3503 = local write "Total No. of Tests"(w4605) -> ()
            n3504 = Decimal String To Number(string=w4604) -> (number=w4608:i32)  [unwired: 2 in, 1 out]
            n3505 = local write "SEN.RUN HRS"(w4608) -> ()
          }
        }
        n3506 = case shown="True" w4599 {
          frame False {
          }
          frame True {
            n3507 = Equal?(x="FLAG 4", y=0.0) -> (x = y?=w4612:bool)
            n3508 = case shown="False" w4612 {
              frame False {
                n3509 = Get Date/Time In Seconds() -> (seconds since 1Jan1904=w4618:timestamp)
                n3510 = local read "START 3"() -> (w4616:dbl)
                n3511 = To Double Precision Float(number=w4618) -> (double precision float=w4617:dbl)
                n3512 = Subtract(x=w4617, y=w4616) -> (x-y=→"SENSOR TIME":dbl)
              }
              frame True {
                n3513 = Get Date/Time In Seconds() -> (seconds since 1Jan1904=w4620:timestamp)
                n3514 = local write "FLAG 4"(100.0 ("FLAG")) -> ()
                n3515 = To Double Precision Float(number=w4620) -> (double precision float=→"START 3":dbl)
              }
            }
          }
        }
        n3516 = local read "Quit"() -> (w4597:bool)
      }
      n3517 = while {
        shift-right: [w4397] -> _
        shift-left: _ -> [w4398]
        tunnel: [w4393] -> _
        i -> [w4393]
        stop <- w4392 stop-if-true
        n3518 = Wait (ms)(milliseconds to wait=u32 50 ("Refresh Rate (ms)")) -> ()  [unwired: 1 out]
        n3519 = local read "Json End Flg"() -> (w4394:bool)
        n3520 = Not(x="Upld AR 2") -> ()  [unwired: 1 out]
        n3521 = local read "Upld AR 2"() -> (w4395:bool)
        n3522 = call "Elapsed Time9"("Time Target (s)"="Sen.Upload Rate (s)", "Reset"=FALSE, "Auto Reset"=TRUE) -> ("Time has Elapsed"=w4404:bool)  [unwired: 9 in, 7 out]
        n3523 = Or(x=w4404, y=w4394) -> (x .or. y?=w4400:bool)
        n3524 = case shown="True" w4400 {
          frame False {
          }
          frame True {
            w4496 = "\"SensorName\":\"" ("string")
            w4466 = " \"},{"
            w4491 = "\",\"SensorState\":\""
            w4493 = "\",\"SensorModelNumber\":\"" ("string")
            w4492 = "\",\"SensorRuntimeHours\":\"" ("string")
            n3525 = local read "model num"() -> (w4490:string[])
            n3526 = local read "Sensor name"() -> (w4509:string[])
            n3527 = local read "run"() -> (w4480:string[])
            n3528 = local read "SENSOR TIME"() -> (w4436:dbl)
            n3529 = local read "out"() -> (w4429:string[])
            n3530 = local read "Total No. of Tests"() -> (w4434:dbl)
            n3531 = Select(t=60.0, s="Run test 3", f=3600.0) -> (s? t:f=w4444:dbl)
            n3532 = Index Array(array=w4490, index #1=1 ("index")) -> (element #1=w4489:string, element #2=w4488:string, element #3=w4487:string, element #4=w4486:string, element #5=w4485:string, element #6=w4484:string)  [unwired: 5 in]
            n3533 = Index Array(array=w4480, index #1=1 ("index")) -> (element #1=w4479:string, element #2=w4478:string, element #3=w4477:string, element #4=w4476:string, element #5=w4475:string, element #6=w4474:string)  [unwired: 5 in]
            n3534 = Index Array(array=w4509, index #1=1 ("index")) -> (element #1=w4508:string, element #2=w4507:string, element #3=w4506:string, element #4=w4505:string, element #5=w4495:string, element #6=w4494:string)  [unwired: 5 in]
            n3535 = Index Array(array=w4429, index #1=1 ("index")) -> (element #1=w4461:string, element #2=w4460:string, element #3=w4459:string, element #4=w4458:string, element #5=w4457:string, element #6=w4456:string)  [unwired: 5 in]
            n3536 = local read "SEN.RUN HRS"() -> (w4432:dbl)
            n3537 = Divide(x=w4436, y=w4444) -> (x/y=w4443:dbl)
            n3538 = Increment(x=w4443) -> (x+1=w4439:dbl)
            n3539 = Number To Decimal String(number=w4439) -> (decimal integer string=→"run hrs":string)  [unwired: 1 in]
            n3540 = Divide(x=w4432, y=3600.0 ("f")) -> (x/y=w4427:dbl)
            n3541 = Round To Nearest(number=w4427) -> (nearest integer value=w4425:dbl)
            n3542 = Number To Decimal String(number=w4425) -> (decimal integer string=w4426:string)  [unwired: 1 in]
            n3543 = Number To Decimal String(number=w4434) -> (decimal integer string=w4435:string)  [unwired: 1 in]
            n3544 = local read "Model No"() -> (w4440:string)
            n3545 = local read "UUID"() -> (w4535:string)
            n3546 = local read "Serial No"() -> (w4539:string)
            n3547 = local read "Secret Key"() -> (w4540:string)
            n3548 = Concatenate Strings("\",\"MachineSerialNumber\":\"" ("string"), w4539) -> (w4543:string)
            n3549 = Concatenate Strings("\",\"ModelNumber\":\"" ("string"), w4440) -> (w4441:string)
            n3550 = Concatenate Strings("\",\"MachineRuntimeHours\":\"" ("string"), w4426) -> (w4544:string)
            n3551 = Concatenate Strings("\",\"MachineRuntimeCycles\":\"", w4435) -> (w4537:string)
            n3552 = Concatenate Strings(w4493, w4489) -> (w4523:string)
            n3553 = Concatenate Strings(w4492, w4479) -> (w4524:string)
            n3554 = Concatenate Strings(w4491, w4461) -> (w4522:string)
            n3555 = Concatenate Strings(w4543, w4441, w4544, w4537) -> (w4546:string)
            n3556 = Concatenate Strings(w4493, w4488) -> (w4520:string)
            n3557 = Concatenate Strings(w4492, w4478) -> (w4519:string)
            n3558 = Concatenate Strings(w4491, w4460) -> (w4521:string)
            n3559 = Concatenate Strings(w4493, w4487) -> (w4515:string)
            n3560 = Concatenate Strings(w4492, w4477) -> (w4516:string)
            n3561 = Concatenate Strings(w4491, w4459) -> (w4514:string)
            n3562 = Concatenate Strings(w4493, w4486) -> (w4512:string)
            n3563 = Concatenate Strings(w4492, w4476) -> (w4511:string)
            n3564 = Concatenate Strings(w4491, w4458) -> (w4513:string)
            n3565 = Concatenate Strings(w4523, w4524, w4522) -> (w4525:string)
            n3566 = Concatenate Strings(w4493, w4485) -> (w4502:string)
            n3567 = Concatenate Strings(w4492, w4475) -> (w4503:string)
            n3568 = Concatenate Strings(w4493, w4484) -> (w4499:string)
            n3569 = Concatenate Strings(w4492, w4474) -> (w4498:string)
            n3570 = Concatenate Strings(w4491, w4457) -> (w4501:string)
            n3571 = Concatenate Strings(w4491, w4456) -> (w4500:string)
            n3572 = Concatenate Strings("{\"SecretKey\":\"", w4540, w4546, "\",\"UUID\" : \"", w4535, "\",\"SensorInformation\":", "[{" ("string")) -> (w4473:string)
            n3573 = Concatenate Strings(w4520, w4519, w4521) -> (w4518:string)
            n3574 = Concatenate Strings(w4515, w4516, w4514) -> (w4517:string)
            n3575 = Concatenate Strings(w4512, w4511, w4513) -> (w4510:string)
            n3576 = Concatenate Strings(w4502, w4503, w4501) -> (w4504:string)
            n3577 = Concatenate Strings(w4499, w4498, w4500) -> (w4497:string)
            n3578 = Concatenate Strings(w4496, w4508, w4525, w4466) -> (w4472:string)
            n3579 = Concatenate Strings(w4496, w4507, w4518, w4466) -> (w4471:string)
            n3580 = Concatenate Strings(w4496, w4506, w4517, w4466) -> (w4470:string)
            n3581 = Concatenate Strings(w4496, w4505, w4510, w4466) -> (w4469:string)
            n3582 = Concatenate Strings(w4496, w4495, w4504, w4466) -> (w4468:string)
            n3583 = Concatenate Strings(w4496, w4494, w4497, "\"}" ("string")) -> (w4467:string)
            n3584 = Concatenate Strings(w4473, w4472, w4471, w4470, w4469, w4468, w4467, "]}" ("string")) -> (w4464:string)
            n3585 = local read "SEN.RUN HRS"() -> (w4431:dbl)
            n3586 = disable-structure shown="Disabled" {
              frame Disabled {
                n3587 = local read "state"() -> (w4550:string[])
                n3588 = Delete From Array(array=w4550, index=0) -> (array with subset deleted=w4548:string[])  [unwired: 1 in, 1 out]
                n3589 = for {
                  N: 6 -> [_]
                  tunnel: w4548 -> [w4561] mode=indexing
                  tunnel: [w4560] -> w4547 mode=indexing
                  n3590 = Equal?(x=w4561, y="Warning") -> (x = y?=w4557:bool)
                  n3591 = Equal?(x=w4561, y="Healthy") -> (x = y?=w4554:bool)
                  n3592 = Select(t="2" ("y"), s=w4557, f="3" ("y")) -> (s? t:f=w4552:string)
                  n3593 = Select(t="1" ("y"), s=w4554, f=w4552) -> (s? t:f=w4560:string)
                }
                "state1" <- w4547
              }
              frame Enabled {
              }
            }
            n3594 = stacked-sequence {
              tunnel: w4464 -> [w4572 _ _]
              tunnel: [_ _ w4588] -> _
              frame #0 {
                (unwired) FALSE ("convert eol (F)")
                w4574 = enum16{"start", "end", "current"}."start" ("pos mode (0:2)")
                n3595 = local read "Path"() -> (w4568:path)
                n3596 = Path To String(path=w4568) -> (string=w4580:string)
                n3597 = Concatenate Strings(w4580, "\\", "Sensor File Name") -> (w4581:string)
                n3598 = local write "standard output 2"(" ") -> ()
                n3599 = String To Path(string=w4581) -> (path=w4571:path)
                n3600 = call <vilib>:"Open_Create_Replace File.vi"("advisory dialog? (display:T)"=FALSE, "function (open:0)"=T25."create or replace", "file path"=w4571) -> ("error out"=w4584:errorcluster, "refnum"=w4583:refnum<file>)  [unwired: 5 in, 2 out]
                n3601 = Set File Position(refnum=w4583, from (0:start)=w4574, error in=w4584) -> (refnum out=w4564:refnum<file>, error out=w4563:errorcluster)  [unwired: 1 in]
                n3602 = Write to Binary File(file (use dialog)=w4564, data=" ", error in=w4563, 5:FALSE ("prepend array or string size? (T)")) -> (refnum out=w4575:refnum<file>, error out=w4576:errorcluster)  [unwired: 2 in, 1 out]
